vi "Subtask 3.vi"() -> ()   [LabVIEW 2016, in "Test.lvrbt"]
uses:
  Test.lvrbt
  <vilib>/NXT/Block Support/NXT_InputPort.ctl
  <vilib>/NXT/Block Support/NXT_OutputPort.ctl
  <vilib>/NXT/Dual Mode Library/Waits/Wait_Num(msec).vi
  <vilib>/NXT/Dual Mode Library/Display/drawText.vi
  <vilib>/NXT/Dual Mode Library/Sensors/EV3_Color_Reflect.vi
  <vilib>/NXT/NXTIO Xnodes/NXTIONodeSubVIs/NXTMotorSteeringOn.vi
  <vilib>/NXT/NXTIO Xnodes/AddressXNode/NXTIOAddress.xnode
  <vilib>/NXT/Subs/LVHSConnector.ctl
  <vilib>/NXT/NXTIO Xnodes/NXTIOXNode/NXTIO.xnode
  <vilib>/NXT/LegoClasses/BrickReference/BrickReference.lvclass
panel:
  out "kD":dbl(graph)
  out "kI":dbl(graph)
  out "kP":sgl(graph)
  out "Combined":dbl(graph)
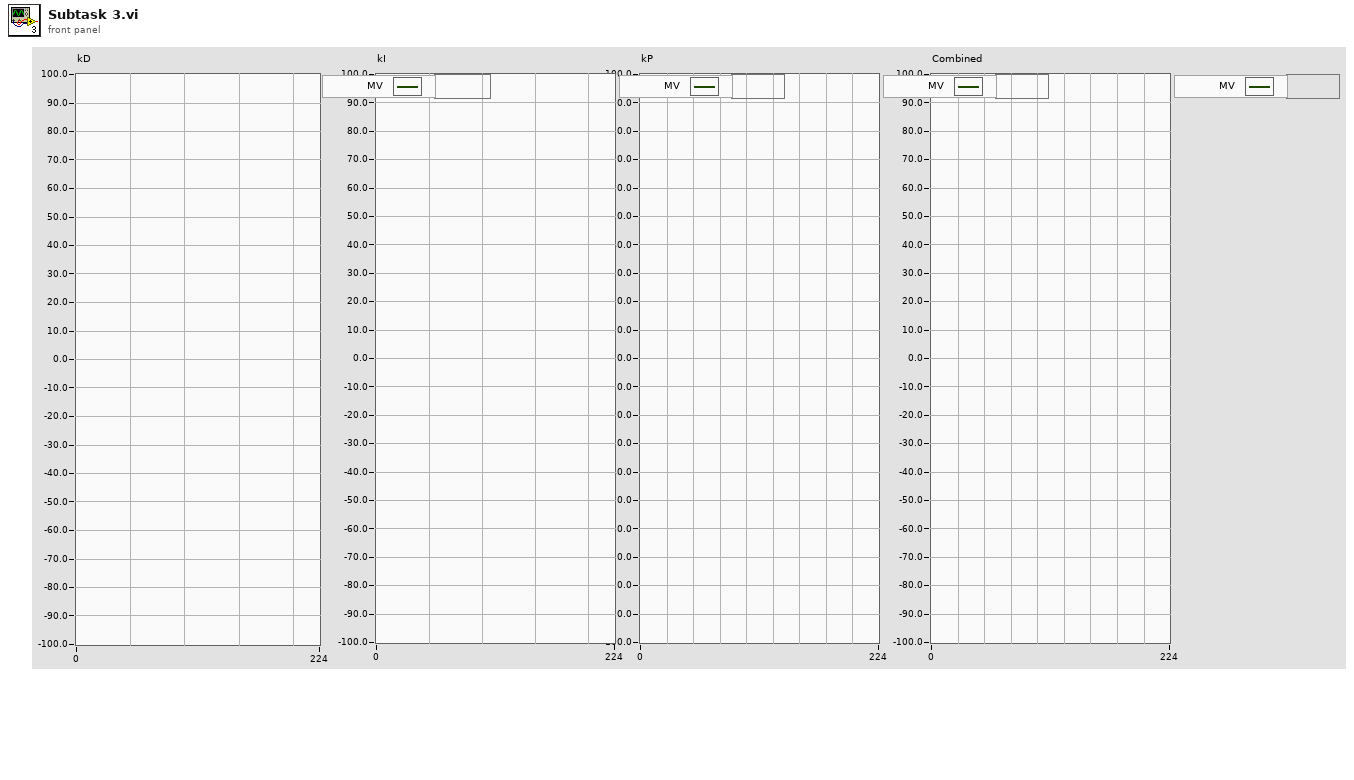
[diagram p1: front panel]
types:
  T1 = typedef "NXT_OutputPort.ctl" = u8
  T2 = typedef "NXT_InputPort.ctl" = u32
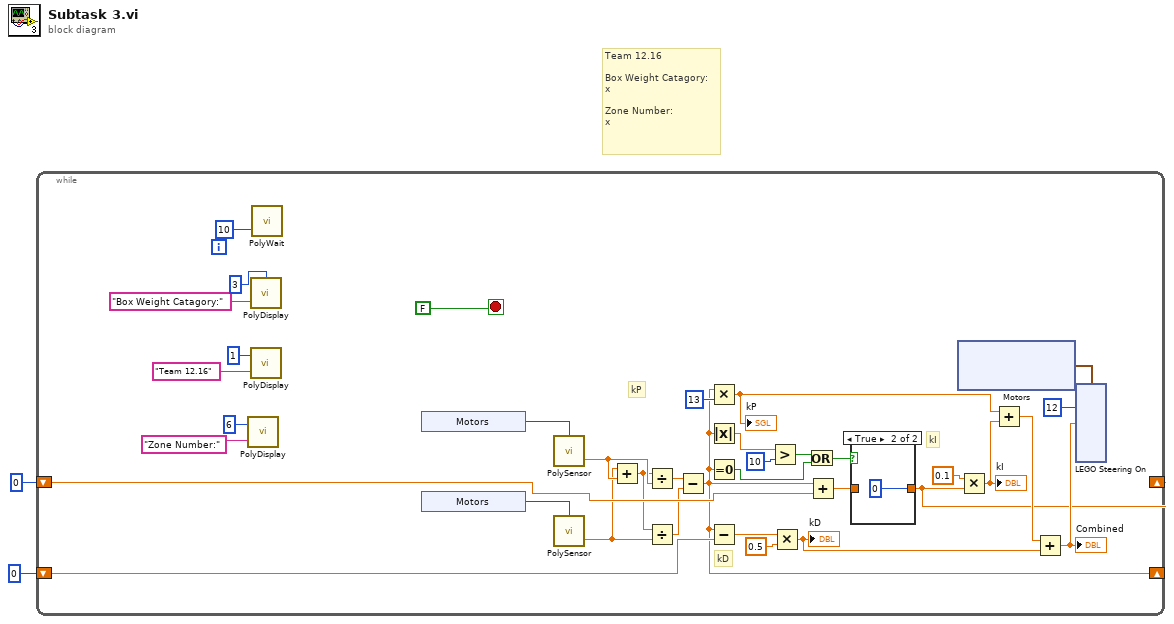
[diagram p0: block diagram]
diagram:
  # "Team 12.16\n\nBox Weight Catagory:\nx\n\nZone Number:\nx"
  n1 = while {
    shift-right: [w14] -> _
    shift-left: 0 -> [w38]
    shift-right: [w15] -> _
    shift-left: 0 -> [w37]
    stop <- FALSE stop-if-true
    # "kD"
    # "kI"
    # "kP"
    n2 = call-poly <vilib>:"PolyDisplay.vi"("Text"="Zone Number:", "Line"=6 ("number")) -> ()  [unwired: 2 in, 1 out]
    n3 = call-poly <vilib>:"PolyDisplay.vi"("Text"="Box Weight Catagory:", "Line"=3 ("number")) -> ()  [unwired: 2 in, 1 out]
    n4 = call-poly <vilib>:"PolyDisplay.vi"("Text"="Team 12.16", "Line"=1 ("number")) -> ()  [unwired: 2 in, 1 out]
    n5 = call-poly <vilib>:"PolyWait.vi"("Time (100 msec)"=u32 10) -> ()  [unwired: 3 in, 1 out]
    n6 = xnode "Motors"() -> ("Sensor"=w12:T2)
    n7 = xnode "Motors"() -> ("Sensor"=w36:T2)
    n8 = call-poly <vilib>:"PolySensor.vi"("Port (Port 1)"=w12) -> ("Scaled Value"=w35:sgl)  [unwired: 2 in, 1 out]
    n9 = call-poly <vilib>:"PolySensor.vi"("Port (Port 1)"=w36) -> ("Scaled Value"=w34:sgl)  [unwired: 2 in, 1 out]
    n10 = Add(x=w34, y=w35) -> (x+y=w33:sgl)
    n11 = Divide(x=w33, y=w35) -> (x/y=w32:sgl)
    n12 = Divide(x=w33, y=w34) -> (x/y=w30:sgl)
    n13 = Subtract(x=w32, y=w30) -> (x-y=w15:sgl)
    n14 = Multiply(x=w15, y=13) -> (x*y=w17:sgl)
    "kP" <- w17
    n15 = Absolute Value(x=w15) -> (abs(x)=w25:sgl)
    n16 = Equal To 0?(x=w15) -> (x = 0?=w27:bool)
    n17 = Subtract(x=w15, y=w37) -> (x-y=w22:sgl)
    n18 = Greater?(x=w25, y=10) -> (0:w24:bool)
    n19 = Multiply(x=w22, y=0.5) -> (x*y=w19:dbl)
    "kD" <- w19
    n20 = Or(x=w24, y=w27) -> (x .or. y?=w26:bool)
    n21 = Add(x=w15, y=w38) -> (x+y=w29:sgl)
    n22 = case shown="True" w26 {
      tunnel: w29 -> [w39 _]
      tunnel: [w39 0] -> w14
      frame False {
      }
      frame True {
      }
    }
    n23 = xnode "Motors"() -> ("Motor"=w5:cluster{"Port":T1, "Port":T1})
    n24 = Multiply(x=0.1, y=w14) -> (x*y=w18:dbl)
    "kI" <- w18
    n25 = Add(x=w17, y=w18) -> (x+y=w20:dbl)
    n26 = Add(x=w20, y=w19) -> (x+y=w16:dbl)
    "Combined" <- w16
    n27 = xnode "LEGO Steering On"("Steering 1"=w16, "Power 1"=12, "Motors"=w5) -> ()  [unwired: 1 in, 1 out]
  }
